vi "Test_Detections.vi"() -> (14 "FugaEn_MIC1":bool, 15 "FugaEn_MIC2":bool, 16 "FugaEn_MIC3":bool, 17 "FugaEn_MIC4":bool, 18 "FugaEn_MIC5":bool, 19 "FugaEn_MIC6":bool)   [LabVIEW 2019]
uses:
  <vilib>/myRIO/Express VI/Onboard IO/DI/DI Express VI.xnode
  <vilib>/myRIO/Instrument Drivers/Onboard IO/DIO/vis/Read.vi
  <vilib>/myRIO/Instrument Drivers/Onboard IO/DIO/DIO.lvlib
  <vilib>/myRIO/Common/Instrument Driver Framework/myRIO v1.0/DIO/typedefs/DIO Channels Enum.ctl
  <vilib>/myRIO/Common/Instrument Driver Framework/myRIO v1.0/DIO/typedefs/DIO Channels List.ctl
  <vilib>/myRIO/Common/Instrument Driver Framework/Utilities/typedefs/Generic FPGA Reference.ctl
  <vilib>/myRIO/Common/Instrument Driver Framework/Utilities/typedefs/myRIO v1.0 Reference.ctl
  <vilib>/myRIO/Common/Instrument Driver Framework/Utilities/typedefs/Hardware Version Enum.ctl
  <vilib>/myRIO/Common/Instrument Driver Framework/Utilities/typedefs/myRIO Generic Hardware Reference.ctl
  <vilib>/myRIO/Instrument Drivers/Onboard IO/DIO/typedefs/DIO Reference.ctl
  <vilib>/myRIO/Instrument Drivers/Onboard IO/DIO/vis/myRIO DIO Open.xnode
  <vilib>/myRIO/Common/Instrument Driver Framework/Utilities/vis/Is FPGA Ref Available.vi
  <vilib>/myRIO/Common/Instrument Driver Framework/myRIO v1.0/DIO/vis/myRIO v1.1 Open DIO.vi
  <vilib>/userDefined/High Color/nirio_resource_hc.ctl
panel:
  in  "Test_MIC4":bool
  in  "Test_MIC5":bool
  in  "Test_MIC6":bool
  in  "Test_MIC3":bool
  in  "Test_MIC2":bool
  in  "Test_MIC1":bool
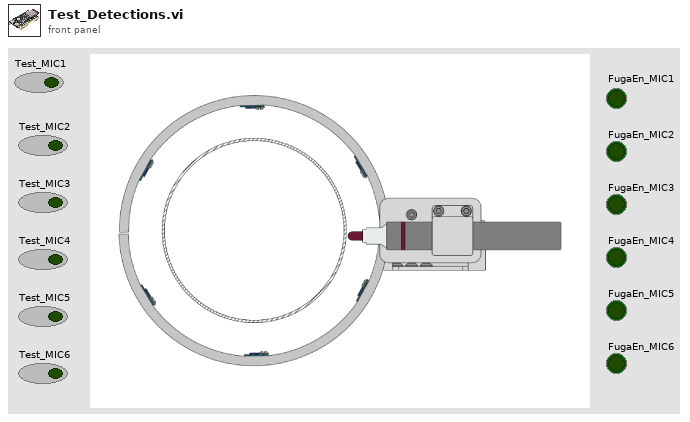
[diagram p1: front panel]
types:
  T1 = typedef "DIO.lvlib/DIO Reference.ctl" = cluster{"myRIO Reference":T2, "DIO Channels List":T6}
  T2 = typedef "myRIO Generic Hardware Reference.ctl" = cluster{"myRIO Model":T3, "myRIO Hardware Reference":T4}
  T3 = typedef "Hardware Version Enum.ctl" = enum16{"Unknown", "myRIO-1900", "myRIO-1950", "roboRIO", "NI ELVIS RIO CM", "ELVIS III"}
  T4 = typedef "myRIO v1.0 Reference.ctl" = cluster{"Generic FPGA Reference":T5, "Allow multiple opens":bool}
  T5 = typedef "Generic FPGA Reference.ctl" = refnum<k20>
  T6 = typedef "DIO Channels List.ctl" = T7[]
  T7 = typedef "DIO Channels Enum.ctl" = enum16{"Not Connected", "C/DIO0", "C/DIO1", "C/DIO2", "C/DIO3", "C/DIO4", "C/DIO5", "C/DIO6", "C/DIO7", "A/DIO0", "A/DIO1", "A/DIO2", "A/DIO3", "A/DIO4", "A/DIO5", "A/DIO6", "A/DIO7", "A/DIO8", "A/DIO9", "A/DIO10", "A/DIO11", "A/DIO12", "A/DIO13", "A/DIO14", "A/DIO15", "A/DIO16", "A/DIO17", "A/DIO18", "A/DIO19", "B/DIO0", "B/DIO1", "B/DIO2", "B/DIO3", "B/DIO4", "B/DIO5", "B/DIO6", "B/DIO7", "B/DIO8", "B/DIO9", "B/DIO10", "B/DIO11", "B/DIO12", "B/DIO13", "B/DIO14", "B/DIO15", "B/DIO16", "B/DIO17", "B/DIO18", "B/DIO19", "LED0", "LED1", "LED2", "LED3", "Button0", "DIO/DIO0", "DIO/DIO1", "DIO/DIO2", "DIO/DIO3", "DIO/DIO4", "DIO/DIO5", "DIO/DIO6", "DIO/DIO7", "DIO/DIO8", "DIO/DIO9", "SPI/CS0", "SPI/CS1", "SPI/CS2", "SPI/CS3", "LED RADIO (Green)", "LED RADIO (Red)", "LED COMM (Green)", "LED COMM (Red)", "LED MODE (Green)", "LED MODE (Red)"}
  T8 = typedef "nirio_resource_hc.ctl" = tag
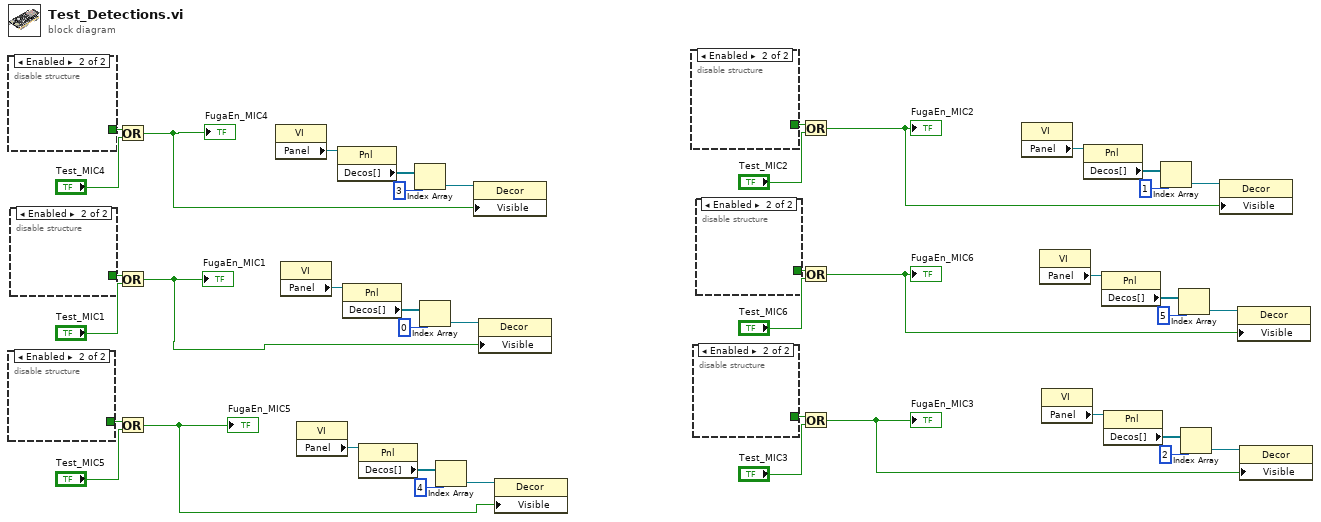
[diagram p0: block diagram]
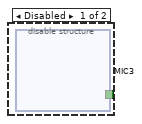
[diagram p2: hidden frame]
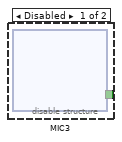
[diagram p3: hidden frame]
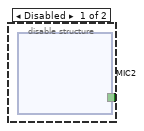
[diagram p4: hidden frame]
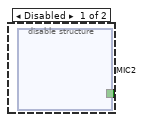
[diagram p5: hidden frame]
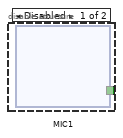
[diagram p6: hidden frame]
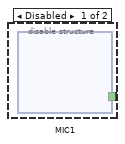
[diagram p7: hidden frame]
diagram:
  n1 = disable-structure shown="Enabled" {
    disable-tunnel: [w43 _] -> w33
    frame Disabled {
      n2 = xnode ("MIC1")() -> ("B/DIO3 (Pin 17)"=w43:bool)  [unwired: 1 in, 1 out]
    }
    frame Enabled {
    }
  }
  n3 = disable-structure shown="Enabled" {
    disable-tunnel: [w79 _] -> w32
    frame Disabled {
      n4 = xnode ("MIC2")() -> ("B/DIO4 (Pin 19)"=w79:bool)  [unwired: 1 in, 1 out]
    }
    frame Enabled {
    }
  }
  n5 = disable-structure shown="Enabled" {
    disable-tunnel: [w115 _] -> w42
    frame Disabled {
      n6 = xnode ("MIC1")() -> ("B/DIO0 (Pin 11)"=w115:bool)  [unwired: 1 in, 1 out]
    }
    frame Enabled {
    }
  }
  n7 = Or(x=w33, y="Test_MIC4") -> (x .or. y?=w27:bool)
  "FugaEn_MIC4" <- w27
  n8 = Or(x=w42, y="Test_MIC1") -> (x .or. y?=w22:bool)
  "FugaEn_MIC1" <- w22
  n9 = Or(x=w32, y="Test_MIC5") -> (x .or. y?=w16:bool)
  "FugaEn_MIC5" <- w16
  n10 = property class="VI"() -> ("Panel"=w30:refnum<vi>)  [unwired: 2 in, 2 out]
  n11 = property class="VI"() -> ("Panel"=w23:refnum<vi>)  [unwired: 2 in, 2 out]
  n12 = property class="VI"() -> ("Panel"=w19:refnum<vi>)  [unwired: 2 in, 2 out]
  n13 = property class="Pnl"(reference=w30) -> ("Decos[]"=w29:refnum<vi>[])  [unwired: 1 in, 2 out]
  n14 = property class="Pnl"(reference=w23) -> ("Decos[]"=w24:refnum<vi>[])  [unwired: 1 in, 2 out]
  n15 = property class="Pnl"(reference=w19) -> ("Decos[]"=w18:refnum<vi>[])  [unwired: 1 in, 2 out]
  n16 = Index Array(array=w29, index=3) -> (element=w28:refnum<vi>)
  n17 = Index Array(array=w24, index=0) -> (element=w25:refnum<vi>)
  n18 = Index Array(array=w18, index=4) -> (element=w17:refnum<vi>)
  n19 = property class="Decor"(reference=w28, "Visible"=w27) -> ()  [unwired: 1 in, 2 out]
  n20 = property class="Decor"(reference=w25, "Visible"=w22) -> ()  [unwired: 1 in, 2 out]
  n21 = property class="Decor"(reference=w17, "Visible"=w16) -> ()  [unwired: 1 in, 2 out]
  n22 = disable-structure shown="Enabled" {
    disable-tunnel: [w151 _] -> w39
    frame Disabled {
      n23 = xnode ("MIC2")() -> ("B/DIO1 (Pin 13)"=w151:bool)  [unwired: 1 in, 1 out]
    }
    frame Enabled {
    }
  }
  n24 = disable-structure shown="Enabled" {
    disable-tunnel: [w187 _] -> w37
    frame Disabled {
      n25 = xnode ("MIC3")() -> ("B/DIO2 (Pin 15)"=w187:bool)  [unwired: 1 in, 1 out]
    }
    frame Enabled {
    }
  }
  n26 = disable-structure shown="Enabled" {
    disable-tunnel: [w223 _] -> w31
    frame Disabled {
      n27 = xnode ("MIC3")() -> ("B/DIO5 (Pin 21)"=w223:bool)  [unwired: 1 in, 1 out]
    }
    frame Enabled {
    }
  }
  n28 = Or(x=w39, y="Test_MIC2") -> (x .or. y?=w11:bool)
  "FugaEn_MIC2" <- w11
  n29 = Or(x=w31, y="Test_MIC6") -> (x .or. y?=w2:bool)
  "FugaEn_MIC6" <- w2
  n30 = Or(x=w37, y="Test_MIC3") -> (x .or. y?=w1:bool)
  "FugaEn_MIC3" <- w1
  n31 = property class="VI"() -> ("Panel"=w12:refnum<vi>)  [unwired: 2 in, 2 out]
  n32 = property class="VI"() -> ("Panel"=w10:refnum<vi>)  [unwired: 2 in, 2 out]
  n33 = property class="VI"() -> ("Panel"=w3:refnum<vi>)  [unwired: 2 in, 2 out]
  n34 = property class="Pnl"(reference=w12) -> ("Decos[]"=w13:refnum<vi>[])  [unwired: 1 in, 2 out]
  n35 = property class="Pnl"(reference=w10) -> ("Decos[]"=w9:refnum<vi>[])  [unwired: 1 in, 2 out]
  n36 = property class="Pnl"(reference=w3) -> ("Decos[]"=w4:refnum<vi>[])  [unwired: 1 in, 2 out]
  n37 = Index Array(array=w13, index=1) -> (element=w14:refnum<vi>)
  n38 = Index Array(array=w9, index=5) -> (element=w8:refnum<vi>)
  n39 = Index Array(array=w4, index=2) -> (element=w5:refnum<vi>)
  n40 = property class="Decor"(reference=w14, "Visible"=w11) -> ()  [unwired: 1 in, 2 out]
  n41 = property class="Decor"(reference=w8, "Visible"=w2) -> ()  [unwired: 1 in, 2 out]
  n42 = property class="Decor"(reference=w5, "Visible"=w1) -> ()  [unwired: 1 in, 2 out]
